vi "latch shoot.vi"() -> (0 "Latch":T1, 1 "Met Requierments for shooting?":bool)   [LabVIEW 2013]
uses:
  typedefs/fg_typedef.ctl
  <vilib>/Rock Robotics/WPI/Solenoid/WPI_SolenoidGetEnum.vi
  <vilib>/Rock Robotics/WPI/Solenoid/WPI_SolenoidValue.ctl
panel:
  # "Acts as a saftey"
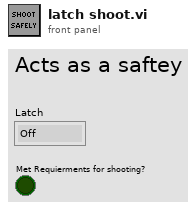
[diagram p1: front panel]
types:
  T1 = typedef "WPI_SolenoidValue.ctl" = enum16{"Off", "On", "Forward", "Reverse"}
  T2 = typedef "fg_typedef.ctl" = enum16{"Get", "Set"}
  T3 = typedef "WPI_DigitalInputDevRef.ctl" = cluster{"DevStatus":errorcluster, "DIO Channel":T4, "Digital Module":T5}
  T4 = typedef "FPGA_DIOChannel.ctl" = enum8{"DIO 1", "DIO 2", "DIO 3", "DIO 4", "DIO 5", "DIO 6", "DIO 7", "DIO 8", "DIO 9", "DIO 10", "DIO 11", "DIO 12", "DIO 13", "DIO 14", "Invalid"}
  T5 = typedef "FPGA_TypedefDigitalModule.ctl" = enum16{"Digital Module 1", "Digital Module 2"}
  T6 = typedef "WPI_SolenoidDevRef.ctl" = cluster{"DevStatus":errorcluster, "Solenoid Module":T7, "Forward Solenoid Channel":T8, "Reverse Solenoid Channel":T8}
  T7 = typedef "FPGA_TypedefSolenoidModule.ctl" = enum16{"Solenoid Module 1", "Solenoid Module 2"}
  T8 = typedef "WPI_SolenoidChannel.ctl" = enum8{"Solenoid 1", "Solenoid 2", "Solenoid 3", "Solenoid 4", "Solenoid 5", "Solenoid 6", "Solenoid 7", "Solenoid 8", "Invalid"}
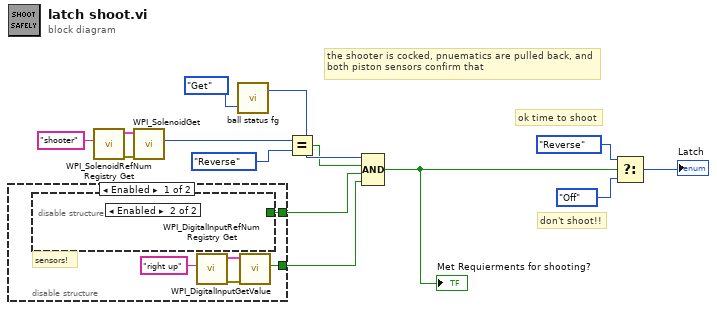
[diagram p0: block diagram]
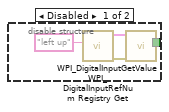
[diagram p2: hidden frame]
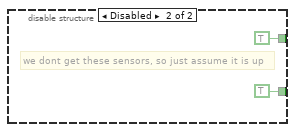
[diagram p3: hidden frame]
diagram:
  # "ok time to shoot"
  # "don't shoot!!"
  # "the shooter is cocked, pnuematics are pulled back, and\nboth piston sensors confirm that"
  n1 = disable-structure shown="Enabled" {
    disable-tunnel: [w18 TRUE ("Value")] -> w9
    disable-tunnel: [w17 TRUE ("Value")] -> w8
    frame Enabled {
      # "sensors!"
      n2 = disable-structure shown="Enabled" {
        disable-tunnel: [w20 _] -> w18
        frame Disabled {
          n3 = call <vilib>:"WPI_DigitalInputRefNum Registry Get.vi"("refnum name"="left up") -> ("error out"=w23:errorcluster, "DigitalInputDevRef"=w22:T3)  [unwired: 9 in]
          n4 = call <vilib>:"WPI_DigitalInputGetValue.vi"("error in (no error)"=w23, "DigitalInputDevRef"=w22) -> ("Value"=w20:bool)  [unwired: 7 in, 2 out]
        }
        frame Enabled {
        }
      }
      n5 = call <vilib>:"WPI_DigitalInputRefNum Registry Get.vi"("refnum name"="right up") -> ("error out"=w19:errorcluster, "DigitalInputDevRef"=w16:T3)  [unwired: 9 in]
      n6 = call <vilib>:"WPI_DigitalInputGetValue.vi"("error in (no error)"=w19, "DigitalInputDevRef"=w16) -> ("Value"=w17:bool)  [unwired: 7 in, 2 out]
    }
    frame Disabled {
      # "we dont get these sensors, so just assume it is up"
    }
  }
  n7 = call <vilib>:"WPI_SolenoidRefNum Registry Get.vi"("refnum name"="shooter") -> ("error out"=w13:errorcluster, "SolenoidDevRef"=w12:T6)  [unwired: 9 in]
  n8 = call-poly <vilib>:"WPI_SolenoidGet.vi"("error in (no error)"=w13, "SolenoidDevRef"=w12) -> ("Value"=w7:T1)  [unwired: 7 in, 2 out]
  n9 = call "ball status fg.vi"("Menu"=fg_typedef."Get") -> ("Ball State"=w10:enum16{"no ball", "holding", "loaded"})  [unwired: 1 out]
  n10 = Equal?(x=w7, y=WPI_SolenoidValue."Reverse") -> (x = y?=w5:bool)
  n11 = Compound Arithmetic op=AND(w10, w5, w9, w8) -> (w2:bool)
  "Met Requierments for shooting?" <- w2
  n12 = Select(t=WPI_SolenoidValue."Reverse" ("y"), s=w2, f=WPI_SolenoidValue."Off" ("y")) -> (s? t:f=→"Latch":T1)
